vi "Flatten .NET Symbol Information.vi"(9 "error in (no error)":errorcluster, 10 ".NET Symbol Information":refnum<k24>) -> (1 "error out":errorcluster, 2 "[.NET Symbol Information]":refnum<k24>[](array[refnum]))   [LabVIEW 2018, in "TwinCAT ADS.lvclass"]
uses:
  TwinCAT ADS.lvclass
  TwinCAT.Ads
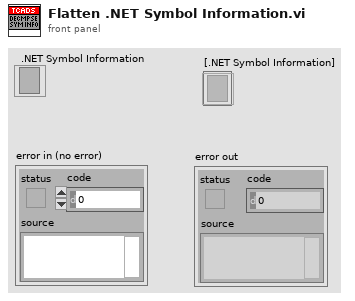
[diagram p1: front panel]
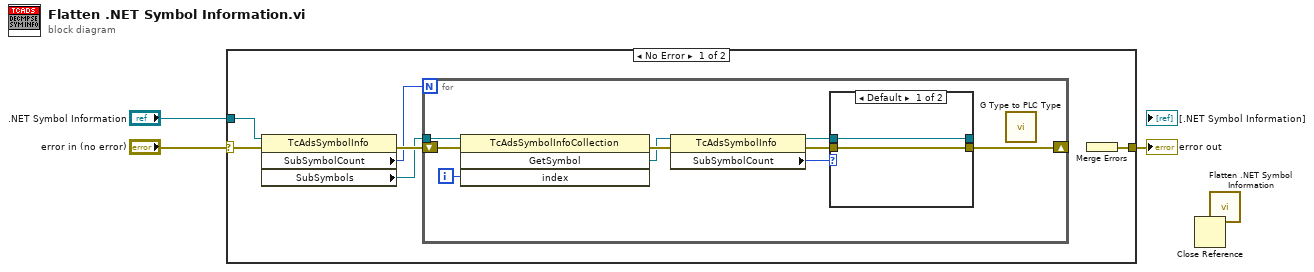
[diagram p0: block diagram]
diagram:
  n1 = case shown="No Error" "error in (no error)" {
    selector: "error in (no error)" -> [w7 w21]
    tunnel: [w9 w21] -> w2
    tunnel: ".NET Symbol Information" -> [w6 _]
    frame No Error {
      n2 = property class="TcAdsSymbolInfo"(reference=w6, error in=w7) -> (error out=w8:errorcluster, "SubSymbolCount"=w5:i32, "SubSymbols"=w4:refnum<k24>)  [unwired: 1 out]
      n3 = for {
        N: w5 -> [_]
        tunnel: w4 -> [w16]
        shift-right: [w10] -> _
        shift-left: w8 -> [w18]
        i -> [w17]
        n4 = invoke class="TcAdsSymbolInfoCollection" method="GetSymbol"(reference=w16, error in=w18, "index"=w17) -> (error out=w15:errorcluster, "GetSymbol"=w14:refnum<k24>)  [unwired: 1 in, 2 out]
        n5 = property class="TcAdsSymbolInfo"(reference=w14, error in=w15) -> (reference out=w11:refnum<k24>, error out=w12:errorcluster, "SubSymbolCount"=w13:i32)
        n6 = case shown="Default" w13 {
          tunnel: w12 -> [w20 _]
          tunnel: w11 -> [w19 _]
          tunnel: [w20 _] -> w10
          tunnel: [w19 _] -> _
          frame Default {
          }
          frame 0 {
          }
        }
        n7 = call "G Type to PLC Type.vi"() -> ()  [unwired: 10 in, 2 out]
      }
      n8 = Merge Errors() -> (w9:errorcluster)  [unwired: 1 in]
    }
    frame Error {
    }
  }
  "error out" <- w2
  n9 = Close Reference() -> ()  [unwired: 2 in, 1 out]
  n10 = call "Flatten .NET Symbol Information.vi"() -> ()  [unwired: 10 in, 2 out]
